vi "Spectrum Move API.vi"(8 "Error In":errorcluster) -> (0 "Error Out":errorcluster)   [LabVIEW 2017]
uses:
  Controls/Command Data [cluster].ctl
  Controls/Commands [enum].ctl
  System Control/System Control Module.lvlib
  UI.lvlib
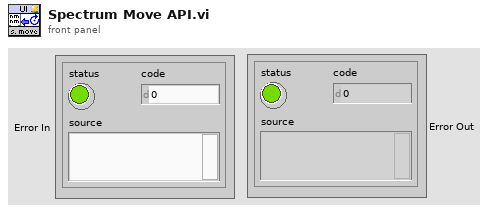
[diagram p1: front panel]
types:
  T1 = typedef "UI.lvlib/Command Data [cluster].ctl" = cluster{"Command":T2, "Data":variant}
  T2 = typedef "UI.lvlib/Commands [enum].ctl" = enum16{"Start", "Spectrum setup", "Spectrum Move", "Move", "Stop"}
  T3 = typedef "System Control Module.lvlib/User Event Refs [cluster].ctl" = cluster{"Stop":refnum<user-event>, "System Error":refnum<user-event>, "UI":refnum<user-event>, "Example Module":refnum<user-event>, "Shutter":refnum<user-event>, "Monochromator":refnum<user-event>}
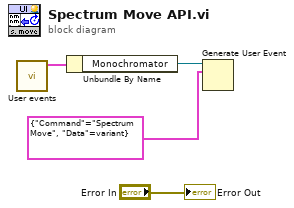
[diagram p0: block diagram]
diagram:
  n1 = call "User events.vi"() -> ("system commands"=w4:T3)  [unwired: 10 in, 1 out]
  n2 = Unbundle By Name(w4) -> ("Monochromator"=w3:refnum<user-event>)
  n3 = Generate User Event(user event=w3, event data cluster=T1 {"Command"=enum."Spectrum Move", "Data"=variant} ("event data")) -> ()  [unwired: 2 in, 2 out]
  "Error Out" <- "Error In"
